vi "setOvenTemperature.vi"(8 "error in (no error)":errorcluster, 10 "temperature":dbl, 11 "OvenController in":refnum<class "OvenController.lvclass">) -> (0 "error out":errorcluster, 3 "OvenController out":refnum<class "OvenController.lvclass">)   [LabVIEW 2023, in "OvenController.lvclass"]
uses:
  OvenController.lvclass
  IDeviceConnection/IDeviceConnection.lvclass
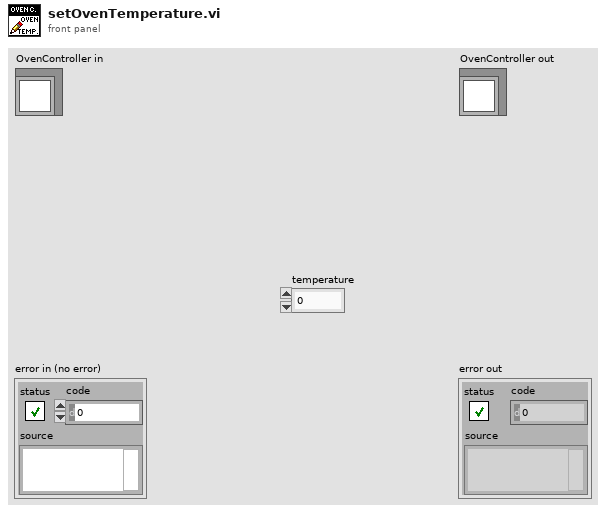
[diagram p1: front panel]
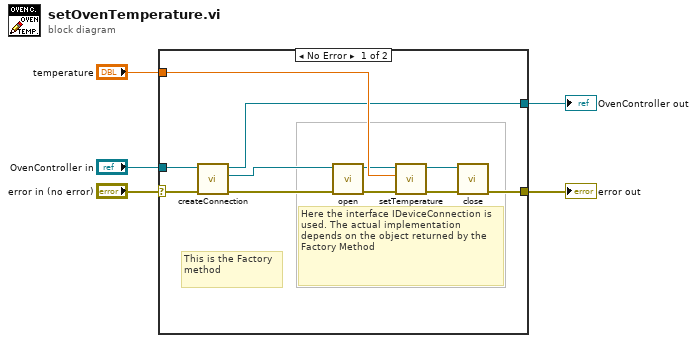
[diagram p0: block diagram]
diagram:
  n1 = case shown="No Error" "error in (no error)" {
    selector: "error in (no error)" -> [w15 w18]
    tunnel: [w6 w18] -> w4
    tunnel: [w12 w17] -> w2
    tunnel: "OvenController in" -> [w14 w17]
    tunnel: "temperature" -> [w13 _]
    frame No Error {
      # "Here the interface IDeviceConnection is used. The actual implementation depends on the object returned by the Factory Method"
      # "This is the Factory method"
      n2 = call-dynamic "createConnection.vi"("error in (no error)"=w15, "OvenController in"=w14) -> ("error out"=w16:errorcluster, "IDeviceConnection"=w10:refnum<class "IDeviceConnection.lvclass">, "OvenController out"=w12:refnum<class "OvenController.lvclass">)  [unwired: 7 in]
      n3 = call-dynamic "open.vi"("error in (no error)"=w16, "IDeviceConnection in"=w10) -> ("error out"=w11:errorcluster, "IDeviceConnection out"=w9:refnum<class "IDeviceConnection.lvclass">)  [unwired: 8 in]
      n4 = call-dynamic "setTemperature.vi"("error in (no error)"=w11, "temperature"=w13, "IDeviceConnection in"=w9) -> ("error out"=w7:errorcluster, "IDeviceConnection out"=w8:refnum<class "IDeviceConnection.lvclass">)  [unwired: 7 in]
      n5 = call-dynamic "close.vi"("error in (no error)"=w7, "IDeviceConnection in"=w8) -> ("error out"=w6:errorcluster)  [unwired: 8 in, 1 out]
    }
    frame Error {
    }
  }
  "error out" <- w4
  "OvenController out" <- w2
